vi "_Read No Objects.vi"(8 "error in (no error)":errorcluster, 11 "Photon Counter SR 400 in":T1={"Mode"=0, "Count Time"=0.0, "Trigger Frequency"=10000000.0, "Trigger External?"=FALSE, "Gate A Mode"=0, "Gate A Width"=0.0, "Gate A Delay"=0.0, "Gate B Mode"=0, "Gate B Width"=0.0, "Gate B Delay"=0.0} {"Mode" items=["A,B For T Preset", "A-B For T Preset", "A+B For T Preset", "A For B Preset"]; "Gate A Mode" items=["CW", "Fixed"]; "Gate B Mode" items=["CW", "Fixed"]}) -> (0 "error out":errorcluster, 2 "4 Data Points":dbl[](array[numeric]), 3 "Photon Counter SR 400 out":T1={"Mode"=0, "Count Time"=0.0, "Trigger Frequency"=10000000.0, "Trigger External?"=FALSE, "Gate A Mode"=0, "Gate A Width"=0.0, "Gate A Delay"=0.0, "Gate B Mode"=0, "Gate B Width"=0.0, "Gate B Delay"=0.0} {"Mode" items=["A,B For T Preset", "A-B For T Preset", "A+B For T Preset", "A For B Preset"]; "Gate A Mode" items=["CW", "Fixed"]; "Gate B Mode" items=["CW", "Fixed"]})   [LabVIEW 2009]
uses:
  Global/GPIB Numbers.vi
  SR400/SR400.lvlib
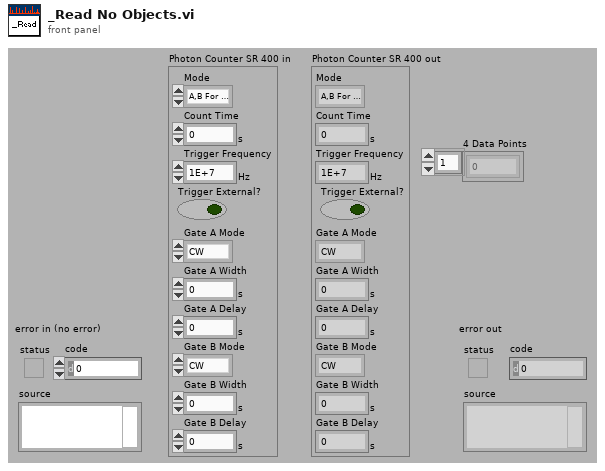
[diagram p1: front panel]
types:
  T1 = cluster{"Mode":u16, "Count Time":dbl[unit], "Trigger Frequency":dbl[unit], "Trigger External?":bool, "Gate A Mode":u16, "Gate A Width":dbl[unit], "Gate A Delay":dbl[unit], "Gate B Mode":u16, "Gate B Width":dbl[unit], "Gate B Delay":dbl[unit]}
  T2 = typedef "GPIB Type Def.ctl" = cluster{"Name":string, "bus":dbl, "GPIB":dbl, "GPIB as string":string, "byte":i32, "VISA Resource Name":refnum<visa-resource-name>}
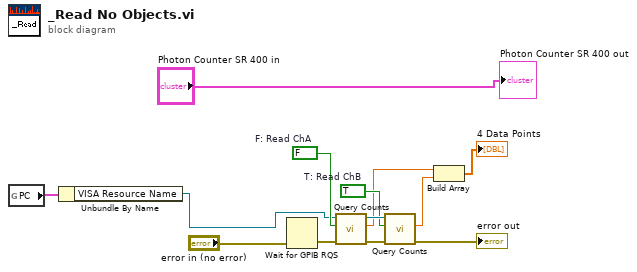
[diagram p0: block diagram]
diagram:
  w10 = TRUE  # T: Read ChB
  w11 = FALSE  # F: Read ChA
  n1 = global read "GPIB Numbers.vi" "PC"() -> (w5:T2)
  n2 = Unbundle By Name(w5) -> ("VISA Resource Name"=w4:refnum<visa-resource-name>)
  n3 = Wait for GPIB RQS(2:"error in (no error)") -> (0:w9:errorcluster)  [unwired: 2 in, 1 out]
  n4 = call "Query Counts.vi"("error in (no error)"=w9, "Read B?"=w11, "VISA resource name"=w4) -> ("error out"=w12:errorcluster, "Counts"=w8:dbl, "VISA resource name out"=w13:refnum<visa-resource-name>)  [unwired: 6 out]
  n5 = call "Query Counts.vi"("error in (no error)"=w12, "Read B?"=w10, "VISA resource name"=w13) -> ("error out"=→"error out":errorcluster, "Counts"=w7:dbl)  [unwired: 7 out]
  n6 = Build Array(w8, w7) -> (→"4 Data Points":dbl[])
  "Photon Counter SR 400 out" <- "Photon Counter SR 400 in"
